vi "Destroy.vi"(8 "Error In":errorcluster, 11 "WebView":refnum<class "WebView.lvclass">) -> (0 "Error Out":errorcluster, 3 "WebView 2":refnum<class "WebView.lvclass">)   [LabVIEW 2024, in "WebView.lvclass"]
uses:
  WebView.lvclass
  WebView.lvclass/WebView.ctl
  <vilib>/sklein/WebView2/Libs/Microsoft.Web.WebView2.Core.dll
  <vilib>/sklein/WebView2/Libs/Microsoft.Web.WebView2.WinForms.dll
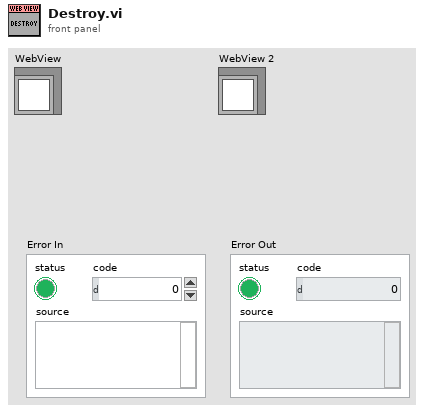
[diagram p1: front panel]
types:
  T1 = typedef "WebView.lvclass/Resources--cluster.ctl" = cluster{"WebView2 Control":refnum<k24>, "Webview2 Core":refnum<k24>, "event callback":refnum<k27>, "Environment":refnum<k24>}
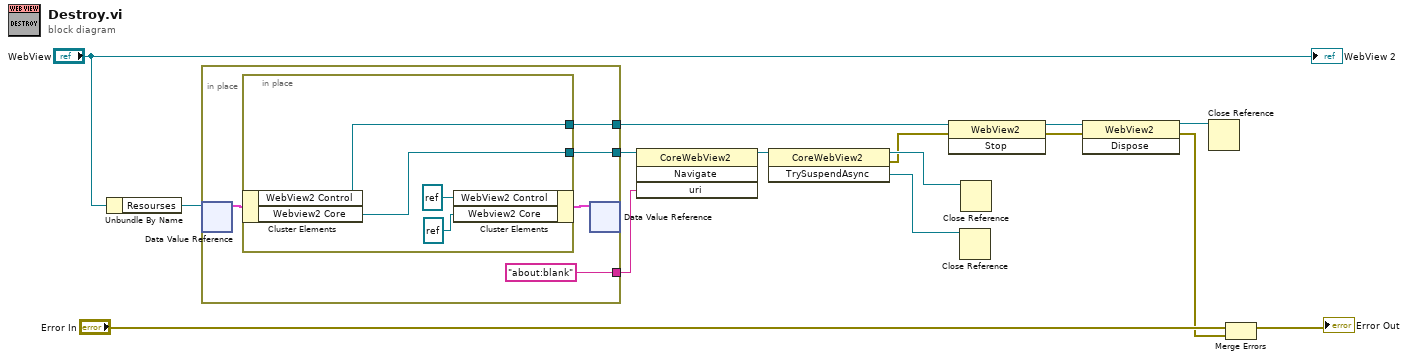
[diagram p0: block diagram]
diagram:
  n1 = Unbundle By Name("WebView") -> ("Resourses"=w9:refnum<data-value>)
  n2 = in-place {
    in-place-border: ["about:blank" ("uri")] -> w11
    in-place-border: [w19] -> w10
    in-place-border: [w16] -> w8
    n3 = in-place-dvr #1(w9) -> (w18:T1)  [unwired: 1 out]
    n4 = in-place {
      in-place-border: [w24] -> w19
      in-place-border: [w22] -> w16
      n5 = in-place-cluster #2(w18) -> ("WebView2 Control"=w22:refnum<k24>, "Webview2 Core"=w24:refnum<k24>)
      n6 = in-place-cluster #2("WebView2 Control"=refnum<k24> refnum ("WebView2"), "Webview2 Core"=refnum<k24> refnum) -> (w17:T1)
    }
    n7 = in-place-dvr #1(w17) -> ()  [unwired: 2 out]
  }
  n8 = invoke class="CoreWebView2" method="Navigate"(reference=w10, "uri"=w11) -> (reference out=w12:refnum<k24>)  [unwired: 2 in, 3 out]
  n9 = invoke class="CoreWebView2" method="TrySuspendAsync"(reference=w12) -> (reference out=w4:refnum<k24>, error out=w3:errorcluster, "TrySuspendAsync"=w5:refnum<k24>)  [unwired: 2 in]
  n10 = invoke class="WebView2" method="Stop"(reference=w8, error in=w3) -> (reference out=w7:refnum<k24>, error out=w6:errorcluster)  [unwired: 1 in, 1 out]
  n11 = Close Reference(reference=w5) -> ()  [unwired: 1 in, 1 out]
  n12 = Close Reference(reference=w4) -> ()  [unwired: 1 in, 1 out]
  n13 = invoke class="WebView2" method="Dispose"(reference=w7, error in=w6) -> (reference out=w2:refnum<k24>, error out=w1:errorcluster)  [unwired: 1 in, 1 out]
  n14 = Close Reference(reference=w2) -> ()  [unwired: 1 in, 1 out]
  n15 = Merge Errors("Error In", w1) -> (→"Error Out":errorcluster)
  "WebView 2" <- "WebView"
